vi "Dummy.vi"(8 "error in (no error)":errorcluster, 10 "Numeric":dbl, 11 "Test Interface Mock In":refnum<class "Test Interface Mock.lvclass">) -> (0 "error out":errorcluster, 2 "Boolean":bool, 3 "Test Interface Mock Out":refnum<class "Test Interface Mock.lvclass">)   [LabVIEW 2020, in "Test Interface Mock.lvclass"]
uses:
  Test Interface Mock.lvclass
  C:/Program Files (x86)/National Instruments/LabVIEW 2020/vi.lib/Astemes/LMock/Responsive Mock.lvclass
  Test Interface Mock.lvclass/Test Interface Mock.ctl
  <vilib>/Astemes/LMock/Responsive Mock.lvclass
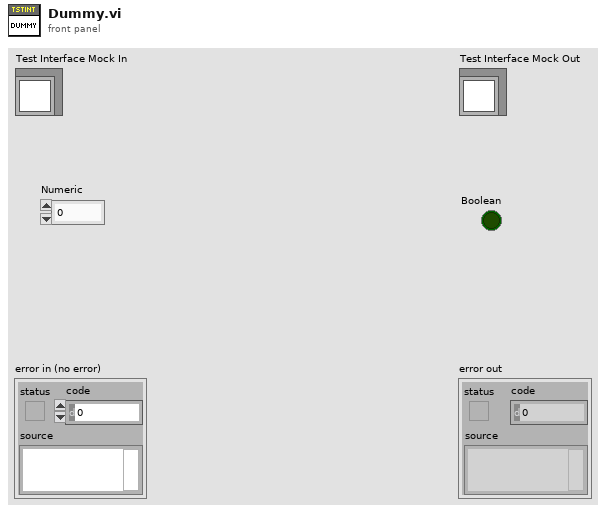
[diagram p1: front panel]
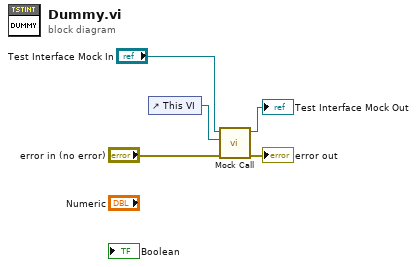
[diagram p0: block diagram]
diagram:
  n1 = control-ref of="This VI"() -> (w3:refnum<vi>)
  n2 = call <vilib>:"Mock Call.vi"("error in (no error)"="error in (no error)", "VI Called"=w3, "Mock In"="Test Interface Mock In") -> ("error out"=→"error out":errorcluster, "Mock Out"=→"Test Interface Mock Out":refnum<class "Test Interface Mock.lvclass">)  [unwired: 7 in]
